vi "lua_error_code_offset.vi"() -> (0 "lua error code offset":i32)   [LabVIEW 2020, in "lua.dll.lvlib"]
uses:
  lua.dll.lvlib
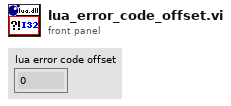
[diagram p1: front panel]
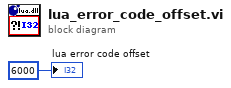
[diagram p0: block diagram]
diagram:
  "lua error code offset" <- 6000 ("lua error code offset")
